vi "get tag counts.vi"(11 "data dictionary in":refnum<class "data bus dictionary.lvclass">) -> (2 "counts":T1[](array[typedef]), 3 "data dictionary out":refnum<class "data bus dictionary.lvclass">)   [LabVIEW 2013, in "data bus dictionary.lvclass"]
doc: "Gets the constitution of the data table, returning an array of types and the associated tag count of each type. If the dictionary is empty, this returns an empty array."
uses:
  data bus dictionary.lvclass
  table/allocation specification.ctl
  tag/Data Type.ctl
  data bus dictionary.lvclass/data bus dictionary.ctl
  tag/data bus tag description.lvclass
  table/data bus values.lvlib
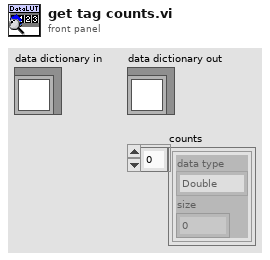
[diagram p1: front panel]
types:
  T1 = typedef "data bus values.lvlib/allocation specification.ctl" = cluster{"data type":T2, "size":i32}
  T2 = typedef "data bus tag description.lvclass/Data Type.ctl" = enum16{"Double", "I64", "Boolean", "Array of Double", "Array of I64", "Variant"}
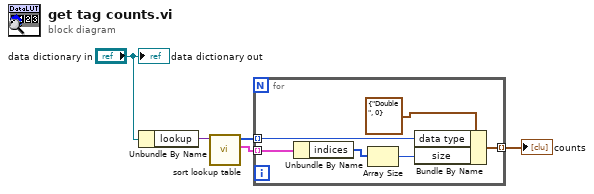
[diagram p0: block diagram]
diagram:
  n1 = Unbundle By Name("data dictionary in") -> ("lookup"=w5:variant)
  n2 = call "sort lookup table.vi"("lookup"=w5) -> ("tags by type"=w2:cluster{"indices":i32[], "names":string[]}[], "types"=w3:T2[])  [unwired: 8 in, 1 out]
  n3 = for {
    tunnel: w3 -> [w8] mode=indexing
    tunnel: w2 -> [w11] mode=indexing
    tunnel: [w6] -> w1 mode=indexing
    n4 = Unbundle By Name(w11) -> ("indices"=w10:i32[])
    n5 = Array Size(array=w10) -> (size(s)=w9:i32)
    n6 = Bundle By Name(cluster=T1 {"data type"=enum."Double", "size"=0} ("allocation"), "data type"=w8, "size"=w9) -> (w6:T1)
  }
  "counts" <- w1
  "data dictionary out" <- "data dictionary in"
